vi "RTS HUT Time Setup.vi"(4 "Third Third":dbl=8.0 format="%#_13g", 5 "Start Index":i32, 6 "Second Third":dbl=6.0 format="%#_13g", 7 "Pre Condition?":bool, 8 "error in (no error)":errorcluster, 9 "First Third":dbl=10.0 format="%#_13g", 11 "Internal Moisture Test (511-B111) - 5 Days":T1 {"Chamber 1-1"."Start Time" format="%<%X\n%x>T"; "Chamber 1-1"."End Time" format="%<%X\n%x>T"; "Chamber 1-2"."Start Time" format="%<%X\n%x>T"; "Chamber 1-2"."End Time" format="%<%X\n%x>T"; "Chamber 1-3"."Start Time" format="%<%X\n%x>T"; "Chamber 1-3"."End Time" format="%<%X\n%x>T"}) -> (0 "error out":errorcluster, 3 "Current Test Output":T1 {"Chamber 1-1"."Start Time" format="%<%X\n%x>T"; "Chamber 1-1"."End Time" format="%<%X\n%x>T"; "Chamber 1-2"."Start Time" format="%<%X\n%x>T"; "Chamber 1-2"."End Time" format="%<%X\n%x>T"; "Chamber 1-3"."Start Time" format="%<%X\n%x>T"; "Chamber 1-3"."End Time" format="%<%X\n%x>T"})   [LabVIEW 2020]
uses:
  Type Definitions/RTS Door Op Data.ctl
  Type Definitions/RTS Door Ops Client.ctl
  Type Definitions/RTS Door Opening Schedule.ctl
  Type Definitions/RTS Door Ops Sequence.ctl
  Type Definitions/RTS Standard Door Opening Test.ctl
panel:
  # "Chamber Conditions:"
  # "Chamber Conditions:"
  # "Chamber Conditions:"
  # "Chamber Conditions:"
  # "Chamber Conditions:"
  # "Chamber Conditions:"
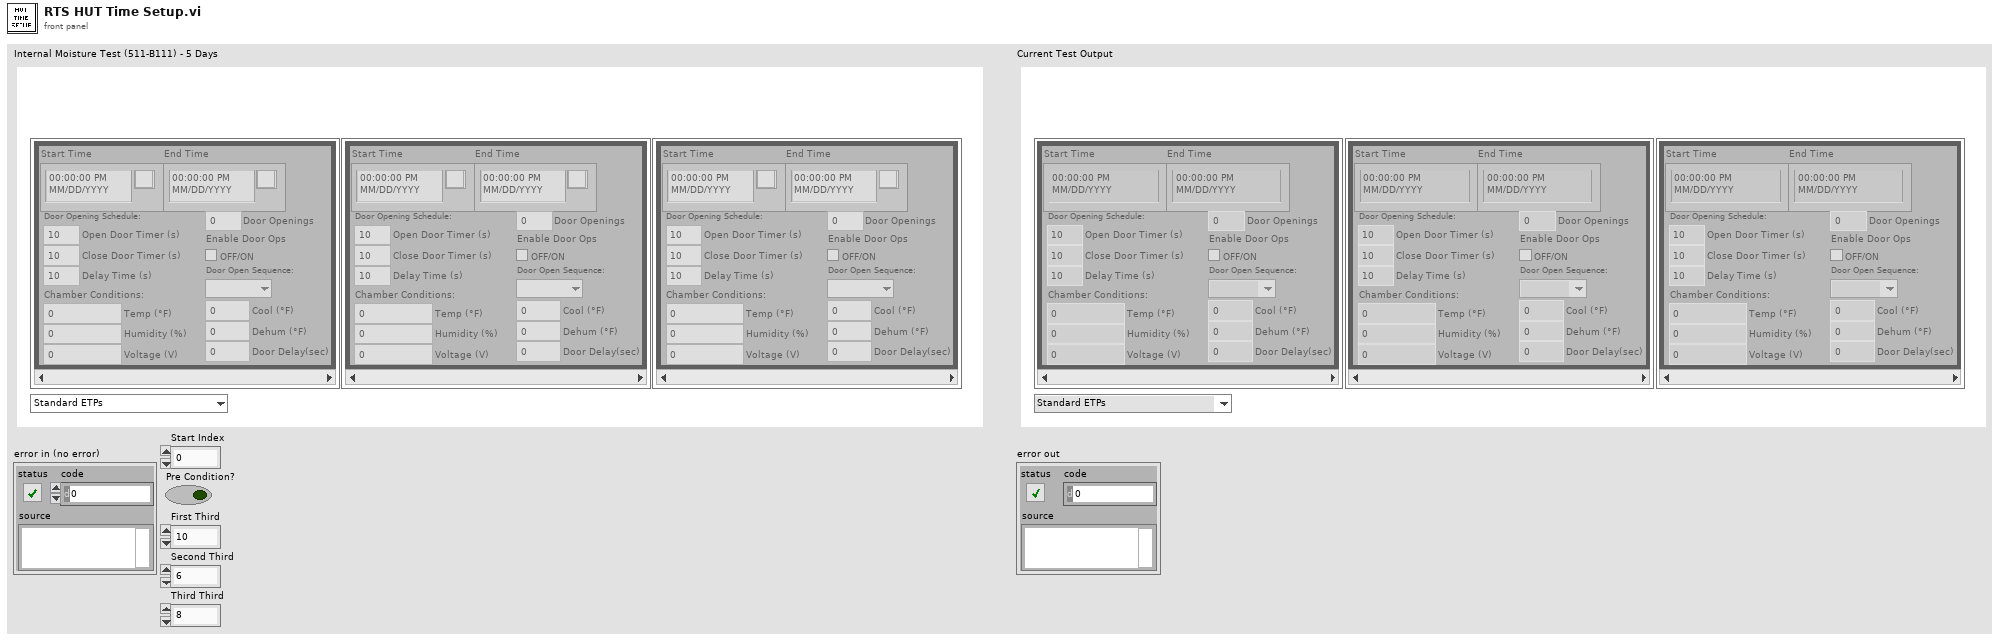
[diagram p1: front panel]
types:
  T1 = typedef "RTS Door Op Data.ctl" = cluster{"Chamber 1-3":T2[], "Chamber 1-2":T2[], "Chamber 1-1":T2[], "Standard Tests 1-1":T5}
  T2 = typedef "RTS Door Ops Client.ctl" = cluster{"End Time":timestamp, "Start Time":timestamp, "Door Opening Schedule:":T3, "Enable Door Ops":bool, "Door Openings":u32, "Temp (°F)":dbl, "Humidity (%)":dbl, "Voltage (V)":dbl, "Door Open Sequence:":T4, "Door Delay(sec)":dbl, "Dehum (°F)":dbl, "Cool (°F)":dbl}
  T3 = typedef "RTS Door Opening Schedule.ctl" = cluster{"Open Door Timer (s)":dbl, "Delay Time (s)":dbl, "Close Door Timer (s)":dbl}
  T4 = typedef "RTS Door Ops Sequence.ctl" = enum16{"", "1st", "2nd", "3rd"}
  T5 = typedef "RTS Standard Door Opening Test.ctl" = enum16{"Standard ETPs", "511-B113 EHUT", "511-B110 HUT", "512-C410 SLAT", "511-B111 Internal Moisture", "511-C401 Moisture Accumulation", "511-B100 No Door Opening (NDO)", "511-B304 ISO Energy Consumption", "Custom Test", "Cancel Test"}
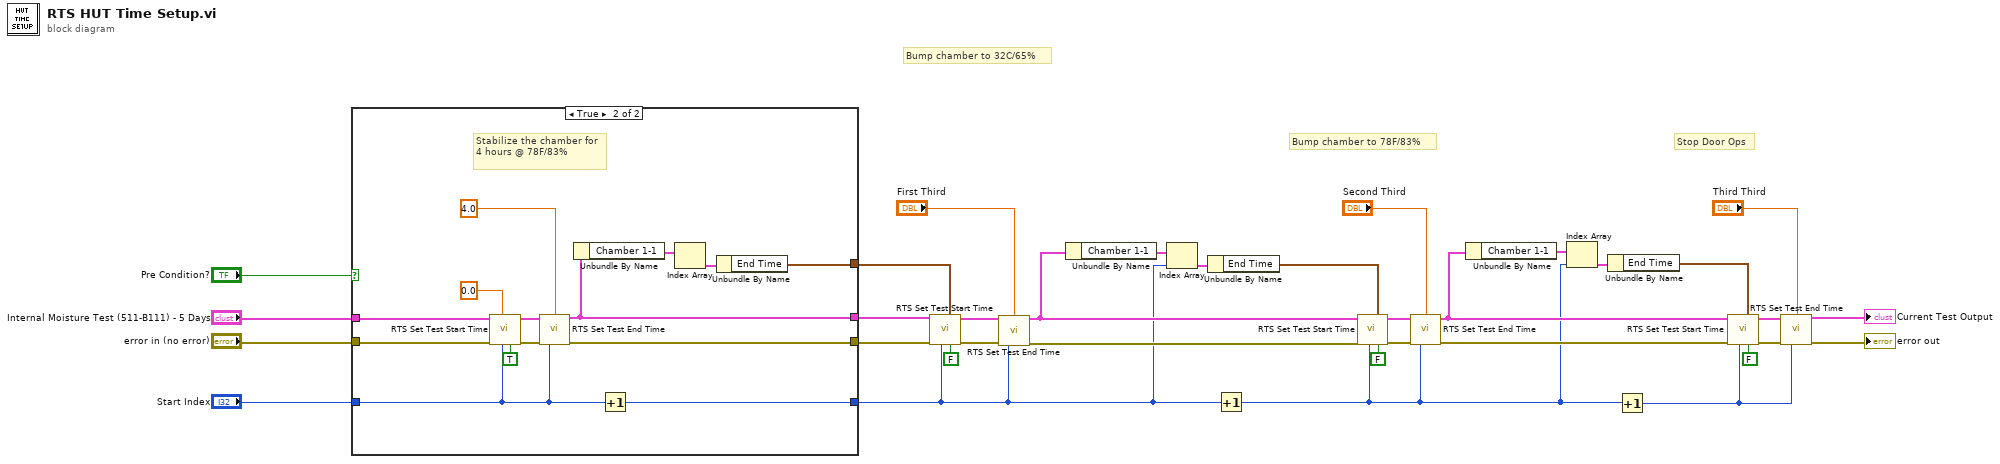
[diagram p0: block diagram]
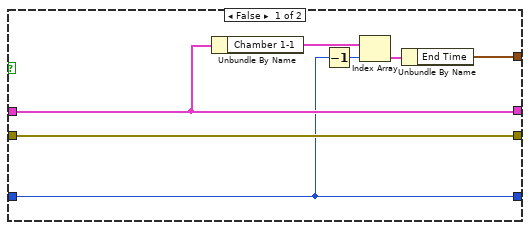
[diagram p2: hidden frame]
diagram:
  # "Stop Door Ops"
  # "Bump chamber to 78F/83%"
  # "Bump chamber to 32C/65%"
  n1 = case shown="True" "Pre Condition?" {
    tunnel: [w39 w54] -> w20
    tunnel: [w38 w51] -> w19
    tunnel: [w37 w48] -> w8
    tunnel: "error in (no error)" -> [w37 w47]
    tunnel: "Internal Moisture Test (511-B111) - 5 Days" -> [w38 w44]
    tunnel: "Start Index" -> [w36 w43]
    tunnel: [w36 w42] -> w4
    frame False {
      n2 = Unbundle By Name(w38) -> ("Chamber 1-1"=w40:T2[])
      n3 = Decrement(x=w36) -> (x-1=w35:i32)
      n4 = Index Array(array=w40, index=w35) -> (element=w41:T2)
      n5 = Unbundle By Name(w41) -> ("End Time"=w39:timestamp)
    }
    frame True {
      # "Stabilize the chamber for\n4 hours @ 78F/83%"
      n6 = call "RTS Set Test Start Time.vi"("Use Current Time As Start?"=TRUE, "index"=w43, "Start Time Offset"=0.0, "Error In"=w47, "Current Test"=w44) -> ("Error Out"=w46:errorcluster, "Current Test Output"=w45:T1)  [unwired: 5 in]
      n7 = call "RTS Set Test End Time.vi"("Current Test"=w45, "Operation Duration (hrs)"=4.0 ("Operation Duration"), "Error In"=w46, "index"=w43) -> ("Current Test Output"=w51:T1, "Error Out"=w48:errorcluster)  [unwired: 10 in]
      n8 = Unbundle By Name(w51) -> ("Chamber 1-1"=w52:T2[])
      n9 = Increment(x=w43) -> (x+1=w42:i32)
      n10 = Index Array(array=w52) -> (element=w53:T2)  [unwired: 1 in]
      n11 = Unbundle By Name(w53) -> ("End Time"=w54:timestamp)
    }
  }
  n12 = call "RTS Set Test Start Time.vi"("Use Current Time As Start?"=FALSE, "Time Start (Gen Prev End)"=w20, "index"=w4, "Error In"=w8, "Current Test"=w19) -> ("Error Out"=w10:errorcluster, "Current Test Output"=w9:T1)  [unwired: 5 in]
  n13 = call "RTS Set Test End Time.vi"("Current Test"=w9, "Operation Duration (hrs)"="First Third", "Error In"=w10, "index"=w4) -> ("Current Test Output"=w24:T1, "Error Out"=w14:errorcluster)  [unwired: 10 in]
  n14 = Unbundle By Name(w24) -> ("Chamber 1-1"=w23:T2[])
  n15 = Index Array(array=w23, index=w4) -> (element=w22:T2)
  n16 = Unbundle By Name(w22) -> ("End Time"=w26:timestamp)
  n17 = Increment(x=w4) -> (x+1=w3:i32)
  n18 = call "RTS Set Test Start Time.vi"("Use Current Time As Start?"=FALSE, "Time Start (Gen Prev End)"=w26, "index"=w3, "Error In"=w14, "Current Test"=w24) -> ("Error Out"=w12:errorcluster, "Current Test Output"=w13:T1)  [unwired: 5 in]
  n19 = call "RTS Set Test End Time.vi"("Current Test"=w13, "Operation Duration (hrs)"="Second Third", "Error In"=w12, "index"=w3) -> ("Current Test Output"=w30:T1, "Error Out"=w17:errorcluster)  [unwired: 10 in]
  n20 = Unbundle By Name(w30) -> ("Chamber 1-1"=w28:T2[])
  n21 = Index Array(array=w28, index=w3) -> (element=w29:T2)
  n22 = Unbundle By Name(w29) -> ("End Time"=w31:timestamp)
  n23 = Increment(x=w3) -> (x+1=w2:i32)
  n24 = call "RTS Set Test Start Time.vi"("Use Current Time As Start?"=FALSE, "Time Start (Gen Prev End)"=w31, "index"=w2, "Error In"=w17, "Current Test"=w30) -> ("Error Out"=w16:errorcluster, "Current Test Output"=w15:T1)  [unwired: 5 in]
  n25 = call "RTS Set Test End Time.vi"("Current Test"=w15, "Operation Duration (hrs)"="Third Third", "Error In"=w16, "index"=w2) -> ("Current Test Output"=→"Current Test Output":T1, "Error Out"=→"error out":errorcluster)  [unwired: 10 in]
